vi "HISTO_READ.vi"(0 "TCP Network Connection in":refnum<k5>, 5 "error in (no error)":errorcluster) -> (14 "TCP Network Connection out":refnum<k5>, 16 "Oscilloscope":u32[](graph), 18 "Status":u8[](array[numeric]), 19 "error out":errorcluster)   [LabVIEW 2019, in "Histogram.lvlib"]
uses:
  Histogram.lvlib
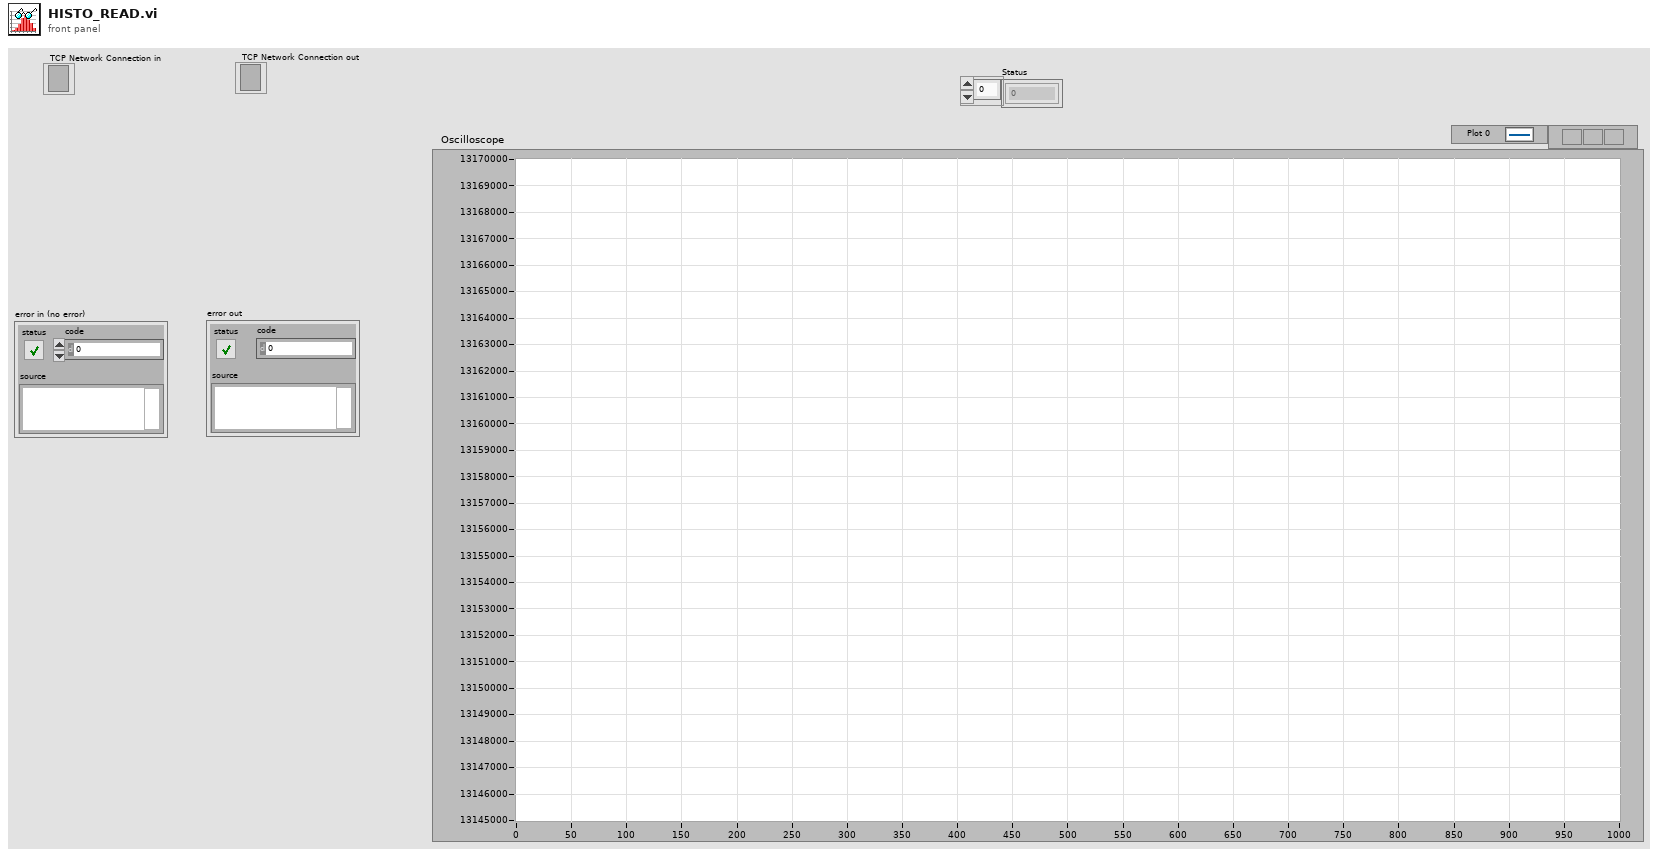
[diagram p1: front panel]
types:
  T1 = enum16{"big-endian, network order", "native, host order", "little-endian"}
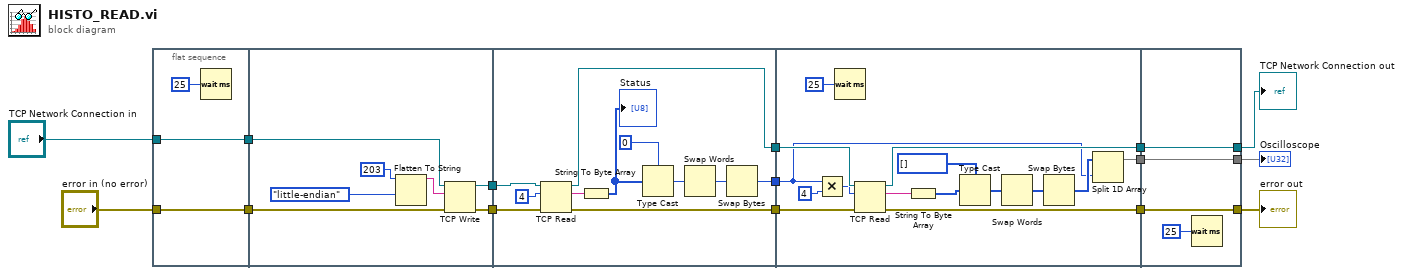
[diagram p0: block diagram]
diagram:
  n1 = flat-sequence {
    tunnel: [w17] -> w11
    tunnel: [w18] -> w10
    tunnel: "error in (no error)" -> [w18]
    tunnel: "TCP Network Connection in" -> [w17]
    tunnel: w11 -> [w25]
    tunnel: w10 -> [w24]
    tunnel: [w23] -> w5
    tunnel: [w22] -> w4
    tunnel: w5 -> [w33]
    tunnel: w4 -> [w36]
    tunnel: [w35] -> w3
    tunnel: [w26] -> w2
    tunnel: [w34] -> w1
    tunnel: w3 -> [w50]
    tunnel: w2 -> [w38]
    tunnel: [w49] -> w8
    tunnel: [w48] -> w7
    tunnel: [w39] -> w6
    tunnel: w1 -> [w51]
    tunnel: [w53] -> w9
    tunnel: [w54] -> w13
    tunnel: [w55] -> w12
    tunnel: w8 -> [w55]
    tunnel: w7 -> [w54]
    tunnel: w6 -> [w53]
    frame #0 {
      n2 = Wait (ms)(milliseconds to wait=u32 25) -> ()  [unwired: 1 out]
    }
    frame #1 {
      n3 = Flatten To String(anything=u32 203 ("element"), byte order (0:big-endian, network order)=T1."little-endian") -> (data string=w19:string)  [unwired: 2 in, 2 out]
      n4 = TCP Write(connection ID=w25, data in=w19, error in (no error)=w24) -> (connection ID out=w23:refnum<k5>, error out=w22:errorcluster)  [unwired: 1 in, 1 out]
    }
    frame #2 {
      n5 = TCP Read(connection ID=w33, bytes to read=4, error in (no error)=w36) -> (connection ID out=w34:refnum<k5>, data out=w32:string, error out=w35:errorcluster)  [unwired: 2 in]
      n6 = String To Byte Array(string=w32) -> (unsigned byte array=w30:u8[])
      "Status" <- w30
      n7 = Type Cast(type=u32 0 ("y"), x=w30) -> (*(type *) &x=w29:u32)
      n8 = Swap Words(1:w29) -> (0:w28:u32)
      n9 = Swap Bytes(anything=w28) -> (byte swapped=w26:u32)
    }
    frame #3 {
      n10 = Multiply(x=w38, y=u32 4) -> (x*y=w46:u32)
      n11 = Wait (ms)(milliseconds to wait=u32 25) -> ()  [unwired: 1 out]
      n12 = TCP Read(connection ID=w51, bytes to read=w46, error in (no error)=w50) -> (connection ID out=w49:refnum<k5>, data out=w37:string, error out=w48:errorcluster)  [unwired: 2 in]
      n13 = String To Byte Array(string=w37) -> (unsigned byte array=w44:u8[])
      n14 = Type Cast(type=u32[] [], x=w44) -> (*(type *) &x=w42:u32[])
      n15 = Swap Words(1:w42) -> (0:w41:u32[])
      n16 = Swap Bytes(anything=w41) -> (byte swapped=w40:u32[])
      n17 = Split 1D Array(array=w40, index=w38) -> (first subarray=w39:u32[])  [unwired: 1 out]
    }
    frame #4 {
      n18 = Wait (ms)(milliseconds to wait=u32 25) -> ()  [unwired: 1 out]
    }
  }
  "error out" <- w13
  "TCP Network Connection out" <- w12
  "Oscilloscope" <- w9
